vi "Utility - Set Pane Origin to 0,0.vi"(8 "error in (no error)":errorcluster, 11 "vi path":path) -> (0 "error out":errorcluster)   [LabVIEW 2014]
uses:
  <vilib>/Utility/miscctls.llb/LVPointTypeDef.ctl
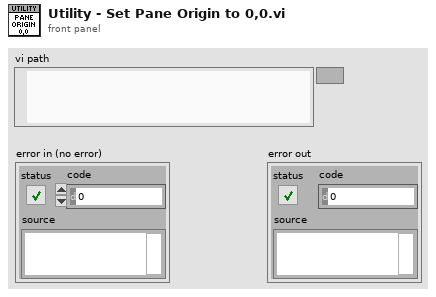
[diagram p1: front panel]
types:
  T1 = typedef "LVPointTypeDef.ctl" = cluster{"Horizontal":i16, "Vertical":i16}
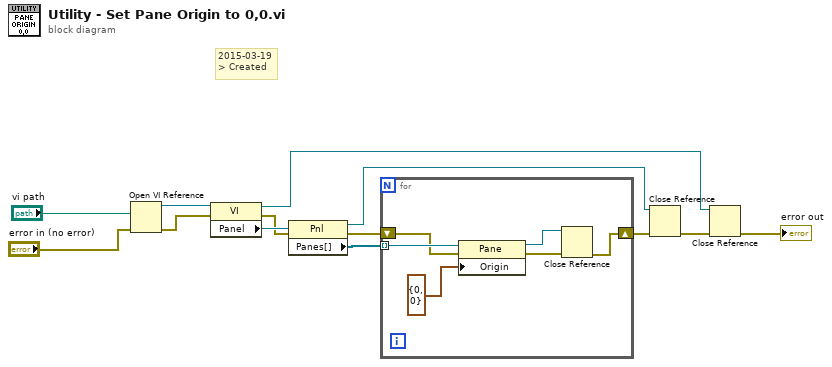
[diagram p0: block diagram]
diagram:
  # "2015-03-19\n> Created"
  n1 = Open VI Reference(vi path="vi path", error in (no error)="error in (no error)") -> (vi reference=w12:refnum<vi>, error out=w9:errorcluster)  [unwired: 4 in]
  n2 = property on="Property Node" class="VI"(reference=w12, error in=w9) -> (reference out=w4:refnum<vi>, error out=w8:errorcluster, "Panel"=w11:refnum<vi>)
  n3 = property on="Property Node" class="Pnl"(reference=w11, error in=w8) -> (reference out=w5:refnum<vi>, error out=w7:errorcluster, "Panes[]"=w10:refnum<vi>[])
  n4 = for {
    tunnel: w10 -> [w19] mode=indexing
    shift-right: [w14] -> w6
    shift-left: w7 -> [w17]
    n5 = property on="Property Node" class="Pane"(reference=w19, error in=w17, "Origin"=T1 {"Horizontal"=0, "Vertical"=0}) -> (reference out=w15:refnum<vi>, error out=w16:errorcluster)
    n6 = Close Reference(reference=w15, error in (no error)=w16) -> (error out=w14:errorcluster)
  }
  n7 = Close Reference(reference=w5, error in (no error)=w6) -> (error out=w3:errorcluster)
  n8 = Close Reference(reference=w4, error in (no error)=w3) -> (error out=→"error out":errorcluster)
